vi "testSetGroupIdx.vi"(8 "error in (no error)":errorcluster) -> (0 "error out":errorcluster)   [LabVIEW 2016]
doc: "Test to set and get index array of Zk and DOF. The sensitivy matrix should be changed at the same time."
uses:
  OptStateEsti/OptStateEsti.lvclass
  StrictDef/InstName.ctl
  OfcFunc.lvlib
  <vilib>/addons/_JKI Toolkits/Caraya/classes/Test/Test.lvclass
  <vilib>/addons/_JKI Toolkits/Caraya/classes/Assert/Assert.lvclass
panel:
  in  "OptStateEsti.lvclass":refnum<class "OptStateEsti.lvclass">
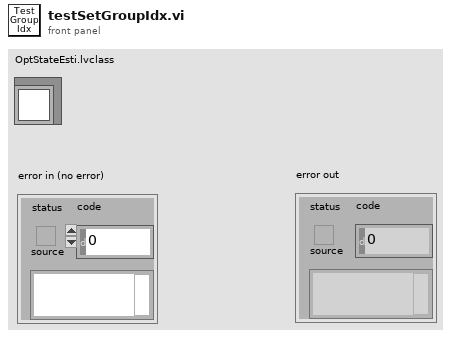
[diagram p1: front panel]
types:
  T1 = cluster{"M2 Hexapod":bool[], "Cam Hexapod ":bool[], "M1M3 Bending Mode":bool[], "M2 Bending Mode":bool[]}
  T2 = typedef "OfcFunc.lvlib/InstName.ctl" = enum16{"lsst", "comcam"}
  T3 = cluster{"Config Dir":path, "Inst Name":T2, "Config File Name":string, "Mapping File Name":string, "Wavelength Table":string, "Intrinc Zk File Name":string, "y2 Corection File Name":string, "Index DOF File Name":string}
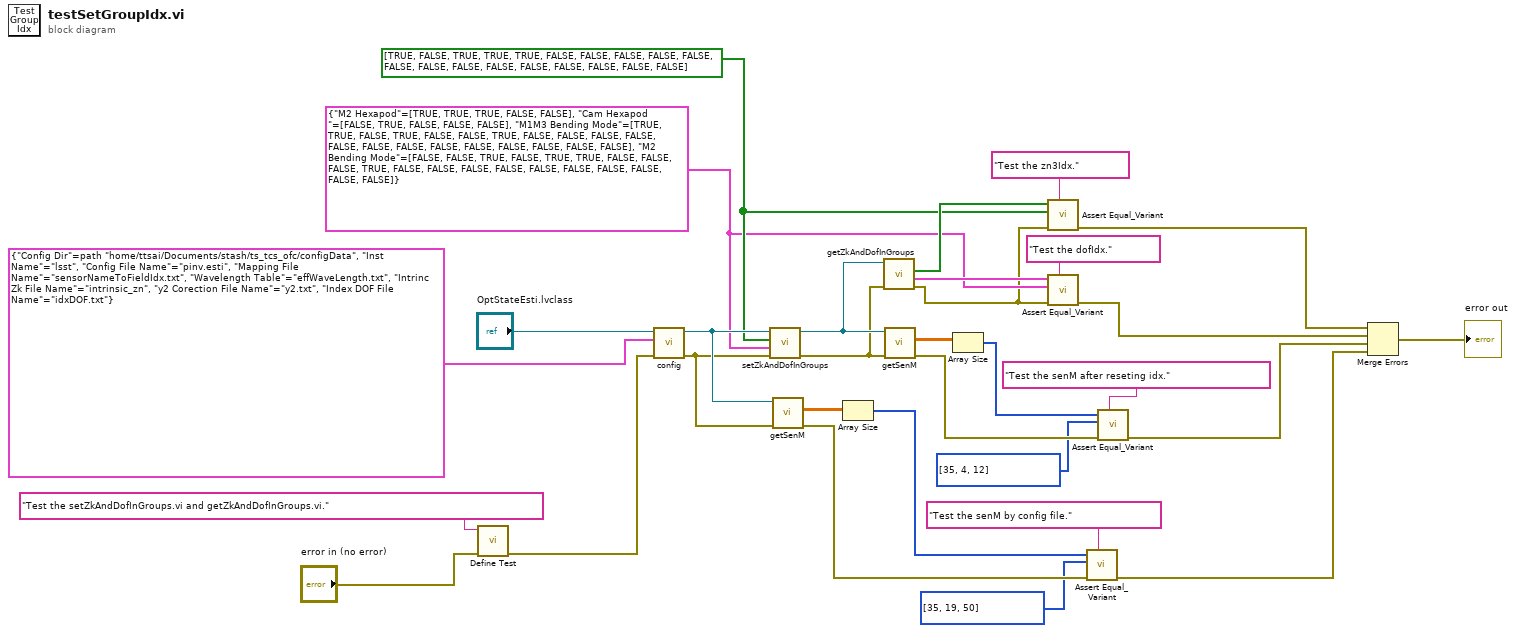
[diagram p0: block diagram]
diagram:
  w16 = T1 {"M2 Hexapod"=[TRUE, TRUE, TRUE, FALSE, FALSE], "Cam Hexapod "=[FALSE, TRUE, FALSE, FALSE, FALSE], "M1M3 Bending Mode"=[TRUE, TRUE, FALSE, TRUE, FALSE, FALSE, TRUE, FALSE, FALSE, FALSE, FALSE, FALSE, FALSE, FALSE, FALSE, FALSE, FALSE, FALSE, FALSE, FALSE], "M2 Bending Mode"=[FALSE, FALSE, TRUE, FALSE, TRUE, TRUE, FALSE, FALSE, FALSE, TRUE, FALSE, FALSE, FALSE, FALSE, FALSE, FALSE, FALSE, FALSE, FALSE, FALSE]} ("DOF in Groups")
  w17 = bool[] [TRUE, FALSE, TRUE, TRUE, TRUE, FALSE, FALSE, FALSE, FALSE, FALSE, FALSE, FALSE, FALSE, FALSE, FALSE, FALSE, FALSE, FALSE, FALSE] ("zn3Idx")
  n1 = call <vilib>:"Define Test.vi"("error in (no error)"="error in (no error)", "Label (VI Title)"="Test the setZkAndDofInGroups.vi and getZkAndDofInGroups.vi.") -> ("error out"=w23:errorcluster)  [unwired: 9 in]
  n2 = call "config.vi"("error in (no error)"=w23, "Configuration"=T3 {"Config Dir"=path "/home/ttsai/Documents/stash/ts_tcs_ofc/configData", "Inst Name"=enum."lsst", "Config File Name"="pinv.esti", "Mapping File Name"="sensorNameToFieldIdx.txt", "Wavelength Table"="effWaveLength.txt", "Intrinc Zk File Name"="intrinsic_zn", "y2 Corection File Name"="y2.txt", "Index DOF File Name"="idxDOF.txt"}, "OptStateEsti in"="OptStateEsti.lvclass") -> ("error out"=w22:errorcluster, "OptStateEsti out"=w29:refnum<class "OptStateEsti.lvclass">)  [unwired: 7 in]
  n3 = call "setZkAndDofInGroups.vi"("error in (no error)"=w22, "DOF in Groups"=w16, "zn3Idx"=w17, "OptStateEsti in"=w29) -> ("error out"=w21:errorcluster, "OptStateEsti out"=w28:refnum<class "OptStateEsti.lvclass">)  [unwired: 6 in]
  n4 = call "getSenM.vi"("error in (no error)"=w22, "OptStateEsti in"=w29) -> ("error out"=w3:errorcluster, "Sen M"=w26:dbl[][][])  [unwired: 7 in, 1 out]
  n5 = Array Size(array=w26) -> (size(s)=w4:i32[])
  n6 = call "getZkAndDofInGroups.vi"("error in (no error)"=w21, "OptStateEsti in"=w28) -> ("error out"=w15:errorcluster, "DOF in Groups"=w18:T1, "zn3Idx"=w19:bool[])  [unwired: 6 in, 1 out]
  n7 = call "getSenM.vi"("error in (no error)"=w21, "OptStateEsti in"=w28) -> ("error out"=w9:errorcluster, "Sen M"=w27:dbl[][][])  [unwired: 7 in, 1 out]
  n8 = Array Size(array=w27) -> (size(s)=w10:i32[])
  n9 = call <vilib>:"Assert Equal_Variant.vi"("Label"="Test the zn3Idx.", "error in (no error)"=w15, "Y"=w17, "X"=w19) -> ("error out"=w14:errorcluster)  [unwired: 7 in]
  n10 = call <vilib>:"Assert Equal_Variant.vi"("Label"="Test the dofIdx.", "error in (no error)"=w15, "Y"=w16, "X"=w18) -> ("error out"=w13:errorcluster)  [unwired: 7 in]
  n11 = call <vilib>:"Assert Equal_Variant.vi"("Label"="Test the senM by config file.", "error in (no error)"=w3, "Y"=i32[] [35, 19, 50], "X"=w4) -> ("error out"=w1:errorcluster)  [unwired: 7 in]
  n12 = call <vilib>:"Assert Equal_Variant.vi"("Label"="Test the senM after reseting idx.", "error in (no error)"=w9, "Y"=i32[] [35, 4, 12], "X"=w10) -> ("error out"=w8:errorcluster)  [unwired: 7 in]
  n13 = Merge Errors(w14, w13, w8, w1) -> (→"error out":errorcluster)
